vi "Api Error Handler.vi"(8 "error in":errorcluster, 11 "HTTP Status":T1) -> (0 "error out":errorcluster)   [LabVIEW 2020, in "InfluxDB v2 Client.lvlib"]
doc: "Error handler for InfluxDB API error codes"
uses:
  InfluxDB v2 Client.lvlib
  HTTP Status.ctl
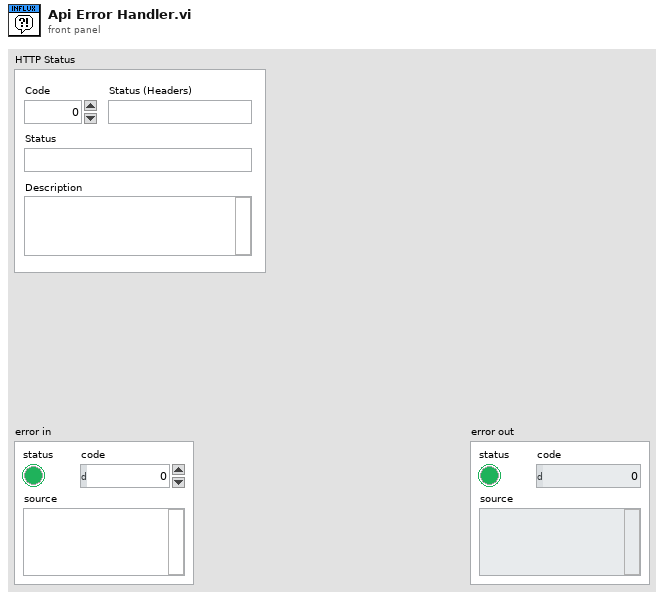
[diagram p1: front panel]
types:
  T1 = typedef "InfluxDB v2 Client.lvlib/HTTP Status.ctl" = cluster{"Code":i32, "Status":string, "Description":string, "Status (Headers)":string}
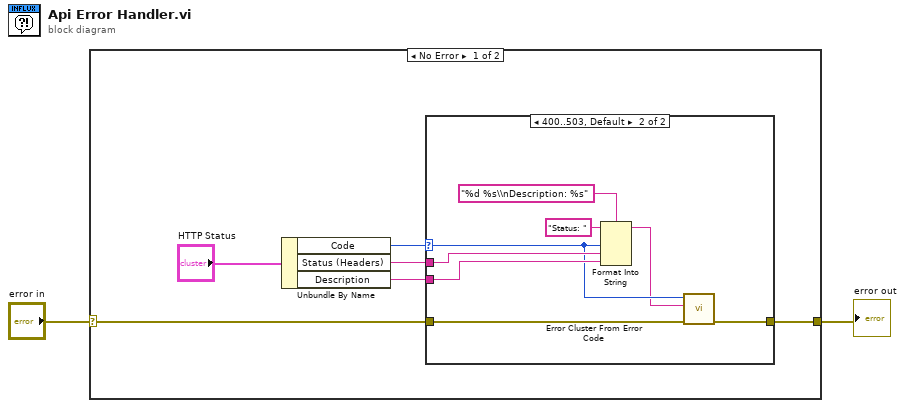
[diagram p0: block diagram]
diagram:
  n1 = case shown="No Error" "error in" {
    selector: "error in" -> [w3 w18]
    tunnel: [w5 w18] -> w1
    frame No Error {
      n2 = Unbundle By Name("HTTP Status") -> ("Code"=w8:i32, "Status (Headers)"=w7:string, "Description"=w6:string)
      n3 = case shown="400..503, Default" w8 {
        selector: w8 -> [_ w12]
        tunnel: w3 -> [w9 w13]
        tunnel: w7 -> [_ w15]
        tunnel: w6 -> [_ w14]
        tunnel: [w9 w10] -> w5
        frame 200, 204 {
        }
        frame 400..503, Default {
          n4 = Format Into String(format string="%d %s\\nDescription: %s", initial string="Status: ", w12, w15, w14) -> (resulting string=w11:string)  [unwired: 1 in, 1 out]
          n5 = call <vilib>:"Error Cluster From Error Code.vi"("error in (no error)"=w13, "error message (\"\")"=w11, "error code (0)"=w12) -> ("error out"=w10:errorcluster)  [unwired: 6 in]
        }
      }
    }
    frame Error {
    }
  }
  "error out" <- w1
